vi "ChannelsGetValues.vi"(10 "Channel paths":string[](array[string])) -> (0 "error out":errorcluster, 1 "Channel Units":string[](array[string]), 2 "Values":dbl[](array[numeric]), 3 "Channels paths out":string[](array[string]))   [LabVIEW 2015, in "ni-veristand-steps-runtime-lib.lvlib"]
uses:
  ni-veristand-steps-runtime-lib.lvlib
  <vilib>/NI Veristand/Execution/Workspace/NI VeriStand - Get Multiple Channel Values.vi
  <vilib>/NI Veristand/Execution/Workspace/NI_VS Workspace ExecutionAPI.lvlib
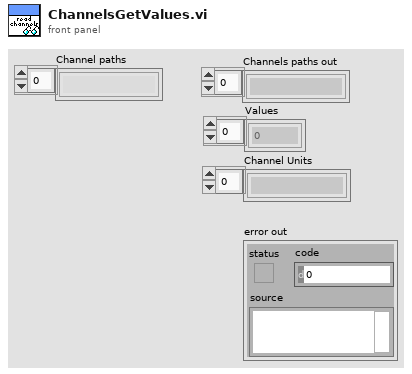
[diagram p1: front panel]
types:
  T1 = typedef "ni-veristand-steps-runtime-lib.lvlib/VeriStand dotNet References.ctl" = cluster{"Project Ref":refnum<k24>, "ModelManager":T2, "AlarmManager":T3, "ChannelFault":T4, "WorkspaceManager":T5}
  T2 = typedef "NI_VS ModelManager ExecutionAPI.lvlib/ModelManagerAPI.ctl" = refnum<k24>
  T3 = typedef "NI_VS AlarmManager ExecutionAPI.lvlib/AlarmManagerAPI.ctl" = refnum<k24>
  T4 = typedef "NI_VS ChannelFault ExecutionAPI.lvlib/ChannelFaultAPI.ctl" = refnum<k24>
  T5 = typedef "NI_VS Workspace ExecutionAPI.lvlib/WorkspaceAPI.ctl" = refnum<k24>
  T6 = typedef "NI_VS Workspace ExecutionAPI.lvlib/NodeInfo.ctl" = cluster{"Name":string, "FullPath":string, "Type":string, "IsChannel":bool, "Channel":cluster{"Unit":string, "Readable":bool, "Writable":bool, "Faultable":bool, "Scalable":bool, "RowDim":u32, "ColumnDim":u32, "Value Table Names":string[], "Value Table Values":dbl[]}, "IsWaveform":bool, "Waveform":cluster{"DataType":T7}}
  T7 = typedef "NI_VS Workspace ExecutionAPI.lvlib/Waveform Data Type.ctl" = enum16{"Double", "ComplexDouble"}
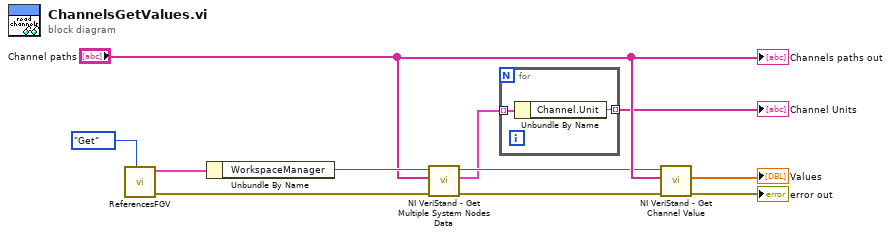
[diagram p0: block diagram]
diagram:
  n1 = call "ReferencesFGV.vi"("Get/Set"=enum16{"Get", "Set"}."Get") -> ("error out"=w6:errorcluster, "VeriStand dotNET Refs out"=w10:T1)  [unwired: 9 in]
  n2 = Unbundle By Name(w10) -> ("WorkspaceManager"=w5:T5)
  n3 = call <vilib>:"NI VeriStand - Get Multiple System Nodes Data.vi"("error in (no error)"=w6, "Node Paths"="Channel paths", "WorkspaceManager in"=w5) -> ("error out"=w7:errorcluster, "Nodes Data"=w2:T6[], "WorkspaceManager out"=w3:T5)  [unwired: 6 in]
  n4 = for {
    tunnel: w2 -> [w13] mode=indexing
    tunnel: [w12] -> w1 mode=indexing
    n5 = Unbundle By Name(w13) -> ("Channel.Unit"=w12:string)
  }
  "Channel Units" <- w1
  n6 = call-poly <vilib>:"NI VeriStand - Get Channel Value.vi"("error in (no error)"=w7, "Channels"="Channel paths", "WorkspaceManager in"=w3) -> ("error out"=→"error out":errorcluster, "Values"=→"Values":dbl[])  [unwired: 6 in, 1 out]
  "Channels paths out" <- "Channel paths"
